vi "Save Raw RP Data.vi"(8 "error in (no error)":errorcluster, 10 "Raw data":string, 11 "RP I-V Driver in":refnum<class "RP I-V Driver.lvclass">) -> (0 "error out":errorcluster, 1 "Finished":bool, 2 "Current read position":i32, 3 "RP I-V Driver out":refnum<class "RP I-V Driver.lvclass">)   [LabVIEW 2016, in "RP I-V Driver.lvclass"]
uses:
  RP I-V Driver.lvclass
  C:/github/NHMFL_Core/Libraries/Instruments/Pulse Driver/Pulse Driver.lvclass
  C:/github/NHMFL_Core/Libraries/Instruments/Instrument Driver/Instrument Driver.lvclass
  Instruments/Pulse Driver/Pulse Driver.lvclass/Pulse Driver.ctl
  Instruments/Instrument Driver/Instrument Driver.lvclass/Instrument Driver.ctl
  Instruments/Pulse Driver/Read Current read position.vi
  Instruments/Pulse Driver/Read tdms file.vi
  Instruments/Instrument Driver/Read Group name.vi
  Instruments/Instrument Driver/Read Channel names.vi
  Instruments/Pulse Driver/Write tdms file.vi
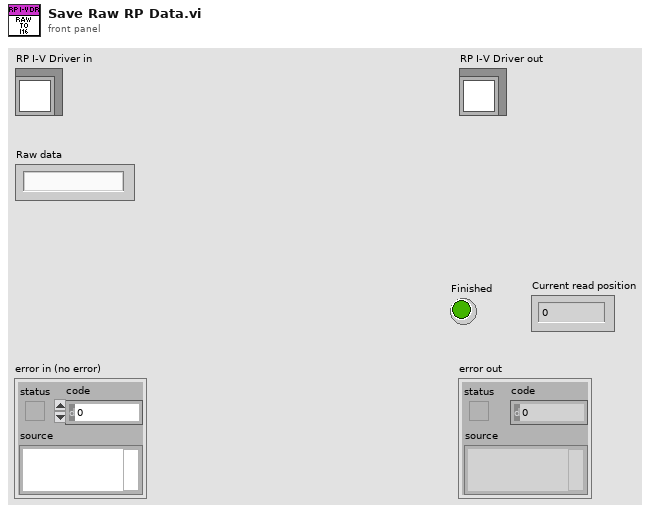
[diagram p1: front panel]
types:
  T1 = enum16{"big-endian, network order", "native, host order", "little-endian"}
  T2 = typedef "RP I-V Configuration.ctl" = cluster{"I-V parameters":T3, "Ranges":dbl[], "Pre-trigger duration":dbl, "Post-trigger duration":dbl, "Output delay":dbl}
  T3 = typedef "I-V parameters.ctl" = cluster{"Start magnitude":dbl, "Magnitude increment":dbl, "End magnitude":dbl, "Ramp length":i32, "Top  length":i32, "Threshold ":dbl, "Processing delay":u16, "Valhalla range":dbl, "Interpolation":i32, "Stop after":u16, "Detector window":i32}
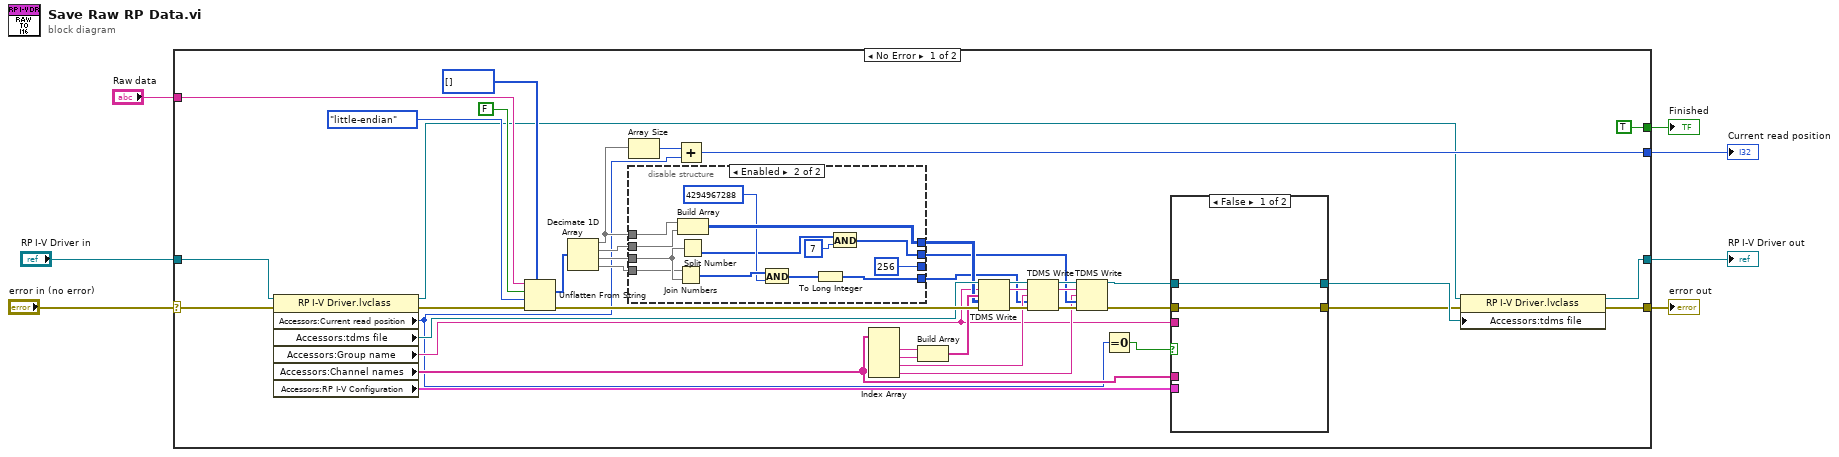
[diagram p0: block diagram]
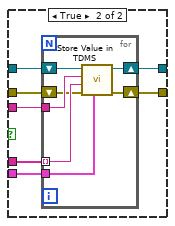
[diagram p2: hidden frame]
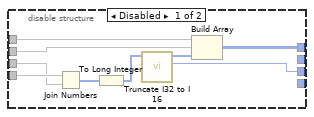
[diagram p3: hidden frame]
diagram:
  n1 = case shown="No Error" "error in (no error)" {
    selector: "error in (no error)" -> [w43 w90]
    tunnel: [w19 w90] -> w4
    tunnel: [w17 w89] -> w6
    tunnel: "RP I-V Driver in" -> [w40 w89]
    tunnel: "Raw data" -> [w45 _]
    tunnel: [w42 _] -> w3
    tunnel: [TRUE ("Finished") _] -> w2
    frame No Error {
      n2 = property class="RP I-V Driver.lvclass"(reference=w40, error in=w43) -> (reference out=w18:refnum<class "RP I-V Driver.lvclass">, error out=w44:errorcluster, "Accessors:Current read position"=w9:i32, "Accessors:tdms file"=w34:refnum<k34>, "Accessors:Group name"=w11:string, "Accessors:Channel names"=w12:string[], "Accessors:RP I-V Configuration"=w10:T2)
      n3 = Unflatten From String(type=i16[] [], binary string=w45, data includes array or string size? (T)=FALSE, byte order (0:big-endian, network order)=T1."little-endian", error in (no error)=w44) -> (value=w46:i16[], error out=w39:errorcluster)  [unwired: 1 out]
      n4 = Decimate 1D Array(w46) -> (w38:i16[], w50:i16[], w35:i16[], w36:i16[])
      n5 = Array Size(array=w38) -> (size(s)=w37:i32)
      n6 = disable-structure shown="Enabled" {
        disable-tunnel: w50 -> [w75 w88]
        disable-tunnel: [w74 w87] -> w30
        disable-tunnel: [w72 256 ("divider")] -> _
        disable-tunnel: w38 -> [w71 w86]
        disable-tunnel: w36 -> [w69 w83]
        disable-tunnel: w35 -> [w68 w84]
        disable-tunnel: [_ w81] -> w25
        disable-tunnel: [_ w76] -> w21
        frame Disabled {
          n7 = Join Numbers(hi=w69, lo=w68) -> ((hi.lo)=w67:u32[])
          n8 = To Long Integer(number=w67) -> (32bit integer=w70:i32[])
          n9 = call "Truncate I32 to I 16.vi"("Data"=w70) -> ("divider"=w72:i32, "Data out"=w73:i16[])  [unwired: 8 in, 1 out]
          n10 = Build Array(w71, w75, w73) -> (w74:i16[][])
        }
        frame Enabled {
          n11 = Join Numbers(hi=w83, lo=w84) -> ((hi.lo)=w82:u32[])
          n12 = Build Array(w86, w88) -> (w87:i16[][])
          n13 = Split Number(x=w84) -> (lo(x)=w78:u8[])  [unwired: 1 out]
          n14 = And(x=w82, y=u32 4294967288) -> (x .and. y?=w80:u32[])
          n15 = To Long Integer(number=w80) -> (32bit integer=w81:i32[])
          n16 = And(x=w78, y=u8 7) -> (x .and. y?=w76:u8[])
        }
      }
      n17 = Add(x=w37, y=w9) -> (x+y=w42:i32)
      n18 = Index Array(array=w12) -> (element #1=w33:string, element #2=w32:string, element #3=w26:string, element #4=w20:string)  [unwired: 4 in]
      n19 = Build Array(w33, w32) -> (w31:string[])
      n20 = TDMS Write(0:w34, 5:w11, 7:w31, 9:w30, 11:w39) -> (4:w28:refnum<k34>, 6:w27:string, 15:w29:errorcluster)  [unwired: 1 in, 1 out]
      n21 = TDMS Write(0:w28, 5:w27, 7:w26, 9:w25, 11:w29) -> (4:w24:refnum<k34>, 6:w23:string, 15:w22:errorcluster)  [unwired: 1 in, 1 out]
      n22 = TDMS Write(0:w24, 5:w23, 7:w20, 9:w21, 11:w22) -> (4:w15:refnum<k34>, 15:w16:errorcluster)  [unwired: 1 in, 2 out]
      n23 = Equal To 0?(x=w9) -> (x = 0?=w8:bool)
      n24 = case shown="False" w8 {
        tunnel: w16 -> [w51 w59]
        tunnel: w15 -> [w52 w58]
        tunnel: [w52 w57] -> w14
        tunnel: [w51 w56] -> w13
        tunnel: w12 -> [_ w55]
        tunnel: w11 -> [_ w54]
        tunnel: w10 -> [_ w53]
        frame False {
        }
        frame True {
          n25 = for {
            tunnel: w55 -> [w63] mode=indexing
            shift-right: [w65] -> w57
            shift-left: w58 -> [w66]
            shift-right: [w60] -> w56
            shift-left: w59 -> [w62]
            tunnel: w54 -> [w64]
            tunnel: w53 -> [w61]
            n26 = call "Store Value in TDMS.vi"("Value"=w61, "Error In"=w62, "channel name"=w63, "group name"=w64, "tdms file"=w66) -> ("Error Out"=w60:errorcluster, "tdms file out"=w65:refnum<k34>)  [unwired: 3 in, 2 out]
          }
        }
      }
      n27 = property class="RP I-V Driver.lvclass"(reference=w18, error in=w13, "Accessors:tdms file"=w14) -> (reference out=w17:refnum<class "RP I-V Driver.lvclass">, error out=w19:errorcluster)
    }
    frame Error {
    }
  }
  "error out" <- w4
  "RP I-V Driver out" <- w6
  "Finished" <- w2
  "Current read position" <- w3
